vi "PH_Powermeter_BaseClass.Read Database.vi"(2 "Instance Name":string, 5 "error in":errorcluster) -> (14 "VISA Resource":string, 15 "Scaling Factor":dbl, 16 "Trigger Level [%]":dbl, 17 "Wavelength [nm]":u32, 18 "Range":u32, 19 "error out":errorcluster)   [LabVIEW 2014, in "PH_Powermeter_BaseClass.lvlib"]
uses:
  PH_Powermeter_BaseClass.lvlib
  PH_Common/PH_Common.lvlib
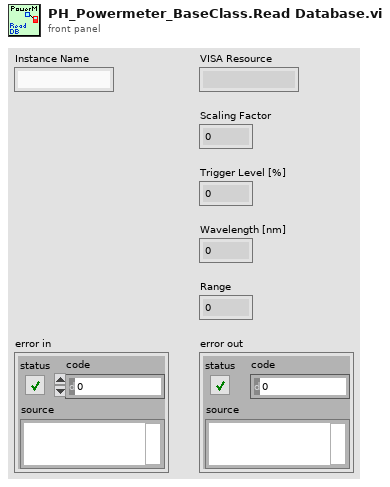
[diagram p1: front panel]
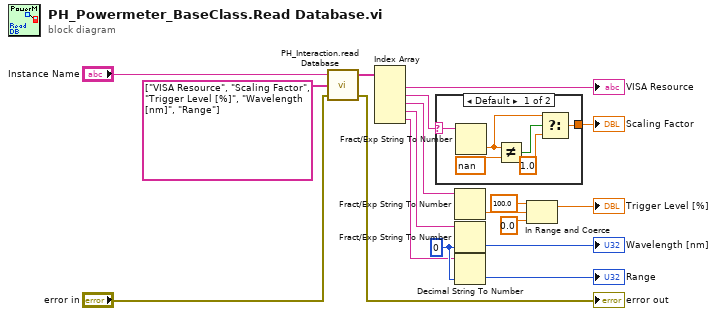
[diagram p0: block diagram]
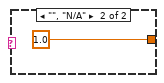
[diagram p2: hidden frame]
diagram:
  w18 = u32 0 ("default (0 DBL)")
  n1 = call "PH_Interaction.read Database.vi"("error in (no error)"="error in", "Strings to search for"=string[] ["VISA Resource", "Scaling Factor", "Trigger Level [%]", "Wavelength [nm]", "Range"], "DB Entry to read"="Instance Name") -> ("error out"=→"error out":errorcluster, "Values"=w8:string[])  [unwired: 1 in]
  n2 = Index Array(array=w8) -> (element #1=→"VISA Resource":string, element #2=w9:string, element #3=w12:string, element #4=w14:string, element #5=w16:string)  [unwired: 5 in]
  n3 = case shown="Default" w9 {
    selector: w9 -> [w24 _]
    tunnel: [w22 1.0 ("Scaling Factor")] -> w5
    frame Default {
      n4 = Fract/Exp String To Number(string=w24) -> (number=w20:dbl)  [unwired: 3 in, 1 out]
      n5 = Not Equal?(x=w20, y=nan) -> (x != y?=w21:bool)
      n6 = Select(t=w20, s=w21, f=1.0) -> (s? t:f=w22:dbl)
    }
    frame "", "N/A" {
    }
  }
  "Scaling Factor" <- w5
  n7 = Fract/Exp String To Number(string=w12) -> (number=w13:dbl)  [unwired: 3 in, 1 out]
  n8 = Fract/Exp String To Number(string=w14, default (0 dbl)=w18) -> (number=→"Wavelength [nm]":u32)  [unwired: 2 in, 1 out]
  n9 = Decimal String To Number(string=w16, default (0L)=w18) -> (number=→"Range":u32)  [unwired: 1 in, 1 out]
  n10 = In Range and Coerce(upper limit=100.0, x=w13, lower limit=0.0) -> (coerced(x)=→"Trigger Level [%]":dbl)  [unwired: 1 out]
